vi "Read Acyclic Frames.vi"(8 "error in":errorcluster, 11 "channel ref in":refnum<k20>) -> (0 "error out":errorcluster, 2 "acyclic frame names":string[](array[string]), 3 "channel ref out":refnum<k20>)   [LabVIEW 2020, in "MIL-STD 1553 Import.lvlib"]
uses:
  MIL-STD 1553 Import.lvlib
  6771c8a3-f311-47c1-9371-f84e0ba0f73c.vi
  3f34854b-cbb0-4767-be42-acd70d4bd91c.vi
  6771c8a3-f311-47c1-9371-f84e0ba0f73c.vi/b1e6fcf8-dac1-42d2-b1fe-151afe06dbd4.vi
  3f34854b-cbb0-4767-be42-acd70d4bd91c.vi/b1e6fcf8-dac1-42d2-b1fe-151afe06dbd4.vi
  Constants.vi
  <vilib>/xml/Get Node Text Content.vi
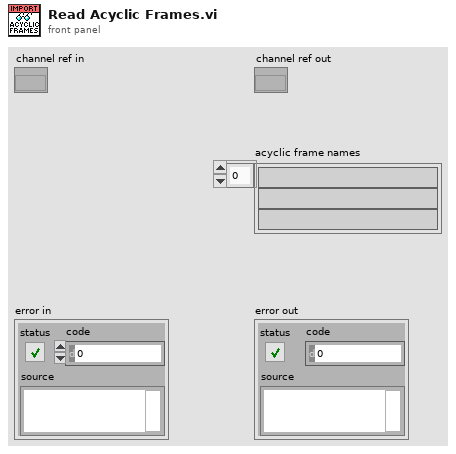
[diagram p1: front panel]
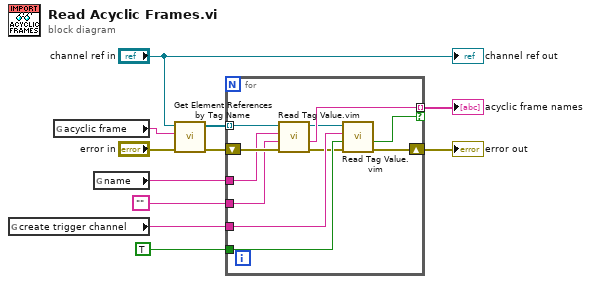
[diagram p0: block diagram]
diagram:
  n1 = global read "Constants.vi" "create trigger channel"() -> (w4:string)
  n2 = global read "Constants.vi" "acyclic frame"() -> (w11:string)
  n3 = global read "Constants.vi" "name"() -> (w6:string)
  n4 = call "Get Element References by Tag Name.vi"("error in"="error in", "tag name"=w11, "node in"="channel ref in") -> ("error out"=w8:errorcluster, "array of elements"=w10:refnum<k20>[])  [unwired: 7 in]
  n5 = for {
    shift-right: [w18] -> w9
    shift-left: w8 -> [w22]
    tunnel: w10 -> [w21] mode=indexing
    tunnel: w6 -> [w20]
    tunnel: "" -> [w19]
    tunnel: w4 -> [w15]
    tunnel: TRUE -> [w16]
    tunnel: [w17] -> w1 mode=indexing if=w12
    n6 = call "Read Tag Value.vim"("error in"=w22, "default"=w19, "tag name"=w20, "node in"=w21) -> ("error out"=w13:errorcluster, "value"=w17:string, "node out"=w14:refnum<k20>)  [unwired: 5 in]
    n7 = call "Read Tag Value.vim"("error in"=w13, "default"=w16, "tag name"=w15, "node in"=w14) -> ("error out"=w18:errorcluster, "value"=w12:bool)  [unwired: 5 in, 1 out]
  }
  "error out" <- w9
  "acyclic frame names" <- w1
  "channel ref out" <- "channel ref in"
